vi "mux2_1(DMM I)_separated.vi"(1 "Boolean array":bool[](array[boolean])=[FALSE, FALSE], 4 "Mem_mapping in":u16[](array[numeric])) -> (8 "Mem_mapping out":u16[](array[numeric]))   [LabVIEW 2018, in "MB Relay.lvlib"]
uses:
  MB Relay.lvlib
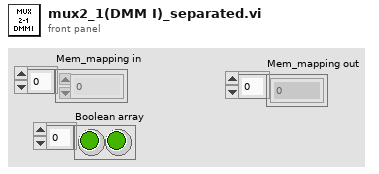
[diagram p1: front panel]
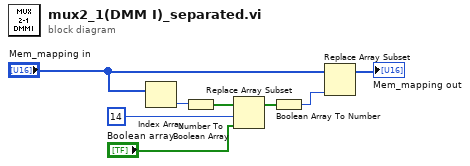
[diagram p0: block diagram]
diagram:
  n1 = Index Array(array="Mem_mapping in") -> (element=w4:u16)  [unwired: 1 in]
  n2 = Number To Boolean Array(number=w4) -> (Boolean array=w3:bool[])
  n3 = Replace Array Subset(array=w3, new element="Boolean array", index=14) -> (w7:bool[])
  n4 = Boolean Array To Number(Boolean array=w7) -> (number=w1:u16)
  n5 = Replace Array Subset(array="Mem_mapping in", new element=w1) -> (→"Mem_mapping out":u16[])  [unwired: 1 in]
